vi "Image.vi"(2 "XRef":refnum<vi>, 3 "State In":T1) -> (0 "Image":picture)   [LabVIEW 2012, in "Foreign Key Sort.xnode"]
uses:
  Foreign Key Sort.xnode
  State.ctl
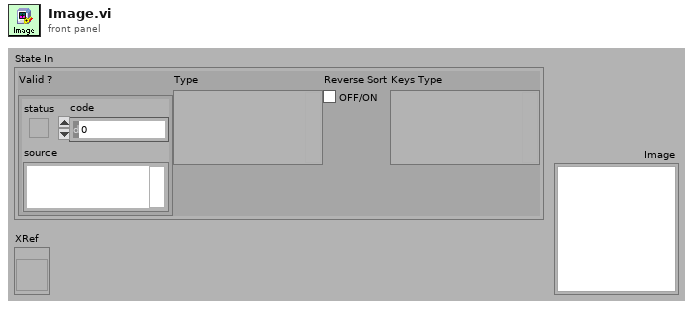
[diagram p1: front panel]
types:
  T1 = typedef "Foreign Key Sort.xnode/State.ctl" = cluster{"Valid ?":errorcluster, "Type":variant, "Reverse Sort":bool, "Keys Type":variant}
  T2 = typedef "imagedata.ctl" = cluster{"image type":i32, "image depth":i32, "image":u8[], "mask":u8[], "colors":u32[], "Rectangle":cluster{"left":i16, "top":i16, "right":i16, "bottom":i16}}
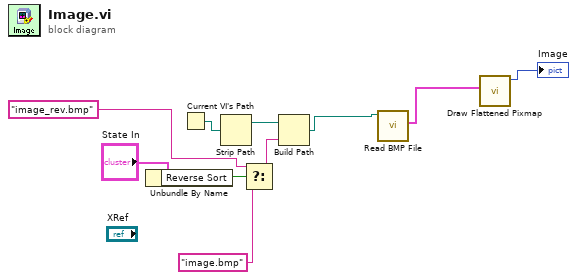
[diagram p0: block diagram]
diagram:
  n1 = Unbundle By Name("State In") -> ("Reverse Sort"=w4:bool)
  n2 = Current VI's Path() -> (path=w9:path)
  n3 = Strip Path(path=w9) -> (stripped path=w8:path)  [unwired: 1 out]
  n4 = Select(t="image_rev.bmp" ("name or relative path"), s=w4, f="image.bmp" ("name or relative path")) -> (s? t:f=w1:string)
  n5 = Build Path(base path=w8, name or relative path=w1) -> (appended path=w7:path)
  n6 = call <vilib>:"Read BMP File.vi"("path to BMP file"=w7) -> ("image data"=w6:T2)  [unwired: 1 in, 9 out]
  n7 = call <vilib>:"Draw Flattened Pixmap.vi"("image data"=w6) -> ("new picture"=→"Image":picture)  [unwired: 1 in, 7 out]
